vi "Delete Session State.vi"(8 "error in (no error)":errorcluster, 11 "Client ID":string) -> (0 "error out":errorcluster)   [LabVIEW 2013, in "MQTT Server.lvlib" / "StoredSessions.lvclass"]
uses:
  StoredSessions.lvclass
panel:
  out "Found?":bool
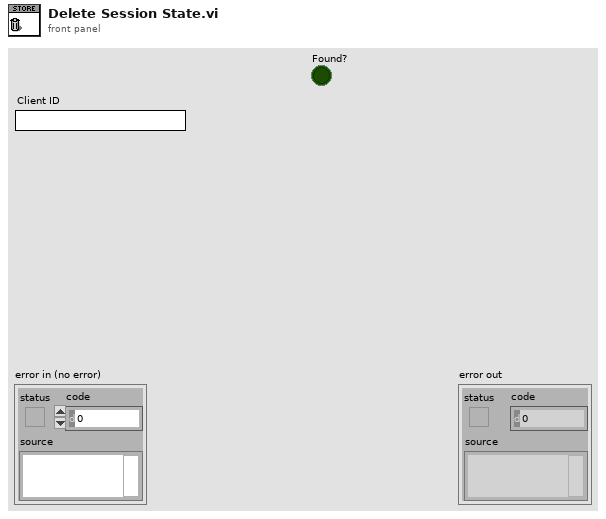
[diagram p1: front panel]
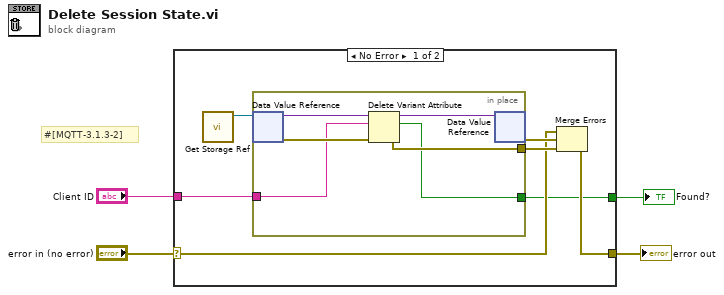
[diagram p0: block diagram]
diagram:
  # "#[MQTT-3.1.3-2]"
  n1 = case shown="No Error" "error in (no error)" {
    selector: "error in (no error)" -> [w7 w18]
    tunnel: [w6 w18] -> w3
    tunnel: "Client ID" -> [w10 _]
    tunnel: [w5 _] -> w1
    frame No Error {
      n2 = call "Get Storage Ref.vi"() -> ("Storage"=w11:refnum<data-value>)  [unwired: 11 in]
      n3 = in-place {
        in-place-border: w10 -> [w13]
        in-place-border: [w16] -> w9
        in-place-border: [w12] -> w5
        n4 = in-place-dvr #1(w11) -> (w14:variant, w15:errorcluster)
        n5 = Delete Variant Attribute(4:w15, 6:w13, 7:w14) -> (0:w16:errorcluster, 2:w12:bool, 3:w17:variant)
        n6 = in-place-dvr #1(w17) -> (w8:errorcluster)  [unwired: 1 out]
      }
      n7 = Merge Errors(w7, w8, w9) -> (w6:errorcluster)
    }
    frame Error {
    }
  }
  "error out" <- w3
  "Found?" <- w1
